vi "NInstrSim_ConfigureWaveformType.appendData2Variant.vi"(0 "initData":variant, 2 "function (0:Sine)":u16(ring) items=["Sine", "Square", "Sine+Noise", "Random", "Chirp"], 5 "error in (no error)":errorcluster) -> (14 "dup initData":variant, 19 "error out":errorcluster)   [LabVIEW 2009, in "HB_Device_Examples.lvlib" / "NInstrSim_ConfigureWaveformType.lvclass"]
doc: "Append initialize data to variant."
uses:
  NInstrSim_ConfigureWaveformType.lvclass
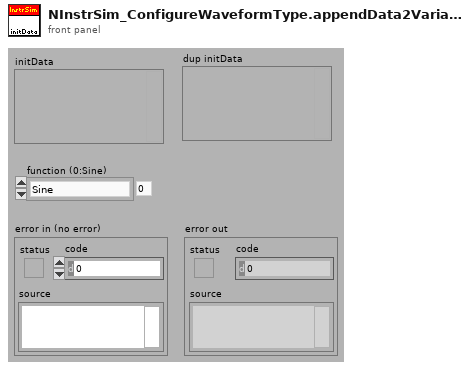
[diagram p1: front panel]
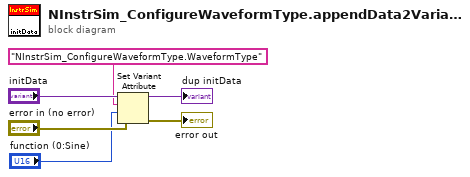
[diagram p0: block diagram]
diagram:
  n1 = Set Variant Attribute(Variant="initData", name="NInstrSim_ConfigureWaveformType.WaveformType", value="function (0:Sine)", error in="error in (no error)") -> (Variant out=→"dup initData":variant, error out=→"error out":errorcluster)  [unwired: 1 out]
